vi "简易流程调试界面.vi"() -> ()   [LabVIEW 2016, in "斯坦道氟化物.lvlib"]
uses:
  <vilib>/Utility/miscctls.llb/LVPointTypeDef.ctl
  <userlib>/_OpenG.lib/array/array.llb/Sort 1D Array (I32)__ogtk.vi
  <vilib>/Plasmionique/MB Master/MB_Master/MB_Master.lvclass
panel:
  in  "调试控件":enum32{"填充流程", "清洗流程", "测试流程", "排空流程", "其他流程"}(tab)
  in  "填充简易流程":i32(listbox)
  in  "清洗简易流程":i32(listbox)
  in  "测试简易流程":i32(listbox)
  in  "排空简易流程":i32(listbox)
  in  "其他简易流程":i32(listbox)
  in  "停止":bool
  in  "单步测试":bool
  out "注射器温度":sgl
  out "消解温度":sgl
  out "ADC":sgl
  out "F3":sgl format="%#.6f"
  out "F2":sgl format="%#.6f"
  out "F1":sgl format="%#.6f"
  out "F0":sgl format="%#.6f"
  in  "启动":bool
  in  "参数下拉列表":u16(ring) items=["总氮"=2]
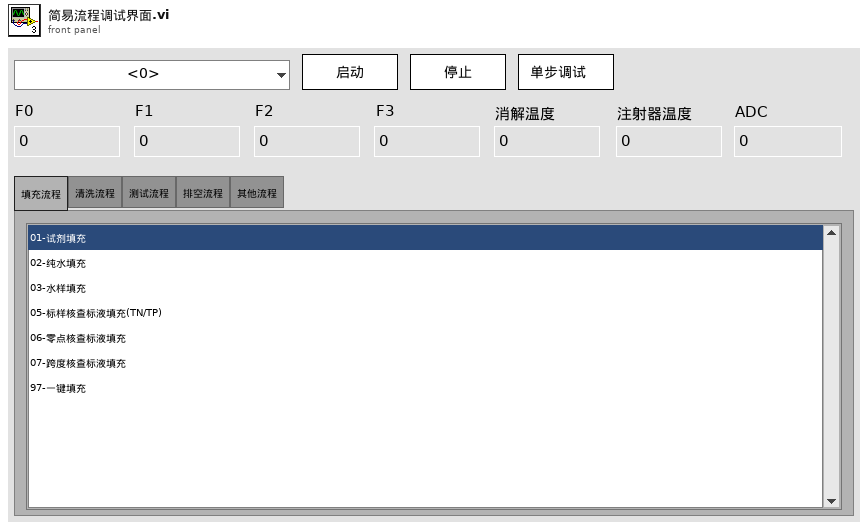
[diagram p1: front panel]
types:
  T1 = typedef "LVPointTypeDef.ctl" = cluster{"Horizontal":i16, "Vertical":i16}
  T2 = typedef "LVRectTypeDef.ctl" = cluster{"Left":i16, "Top":i16, "Right":i16, "Bottom":i16}
  T3 = typedef "LVStringsAndValuesArrayTypeDef_U16.ctl" = cluster{"String":string, "Value":u16}[]
  T4 = typedef "操作日志字段定义.ctl" = cluster{"时间":timestamp, "参数":string, "日志信息":string, "流程参数":string}
  T5 = enum16{"跨度核查", "水样测量", "零点核查", "标样核查", "加标回收", "快捷测试", "空白校准", "标样校准"}
  T6 = cluster{"系统时间":timestamp, "工作状态":u16, "测量模式":enum16{"待机", "连续模式", "周期模式", "定点模式", "受控模式", "手动模式"}, "告警代码":u16, "故障代码":u16, "日志代码":u16, "软件版本":u16, "F0":sgl, "F1":sgl, "F2":sgl, "F3":sgl, "T":sgl, "H":sgl, "id":u16, "flowid":u16, "量程":u16, "总磷控温温度1":sgl, "营养盐控温温度2":sgl, "ADC":sgl}
  T7 = enum32{"Bad", "Idle", "Run top level", "Running"}
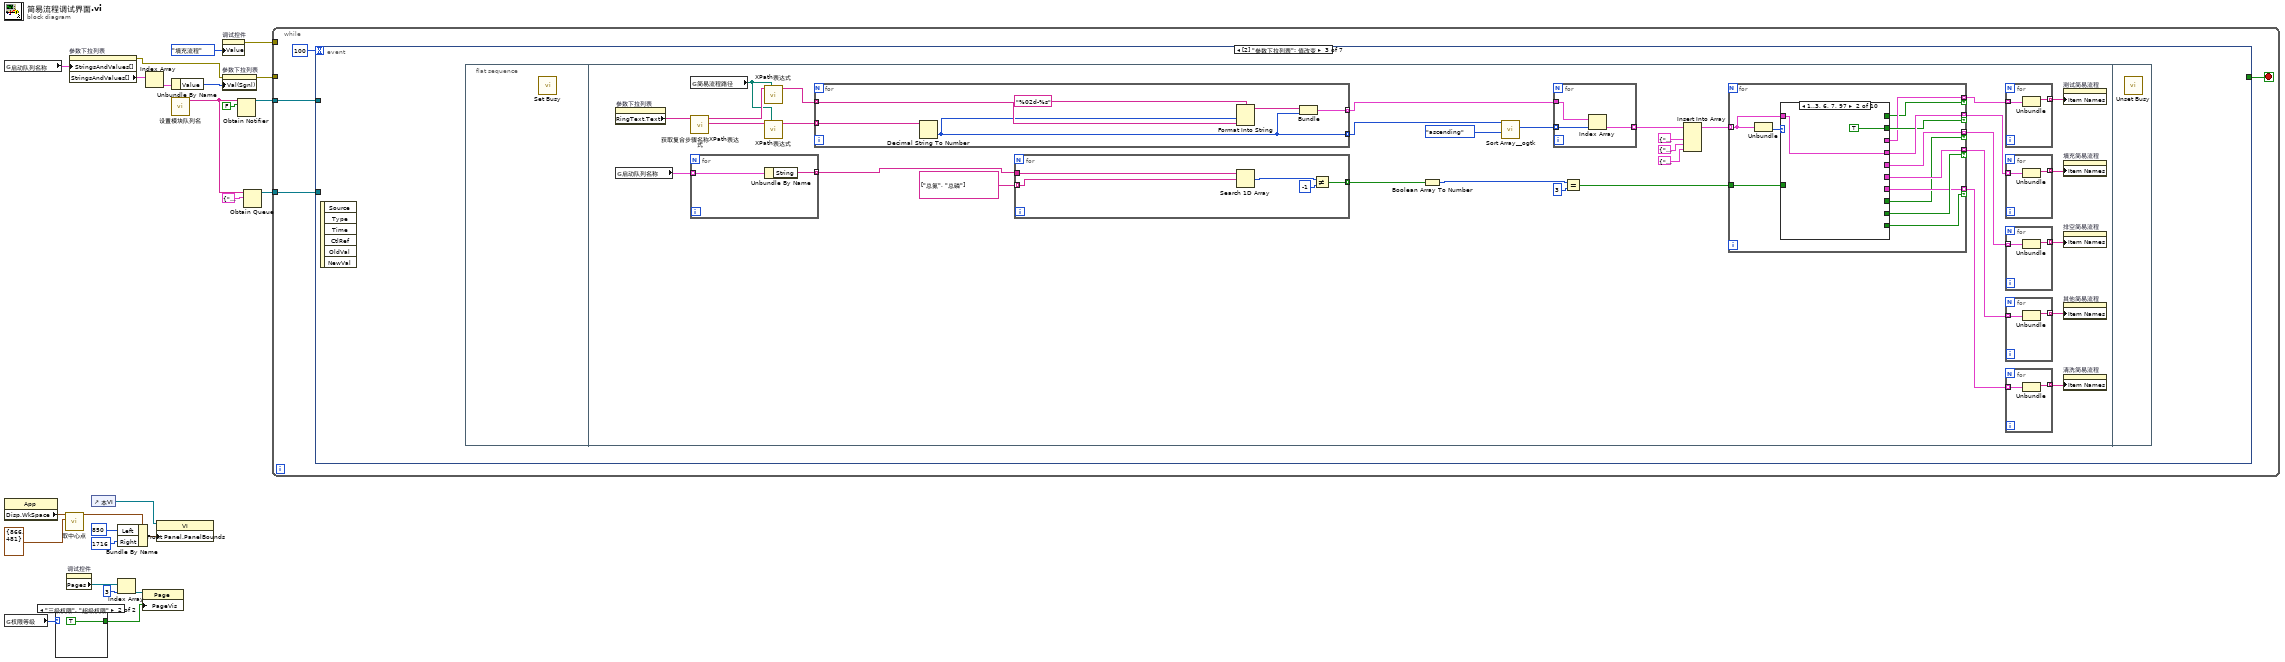
[diagram p0: block diagram]
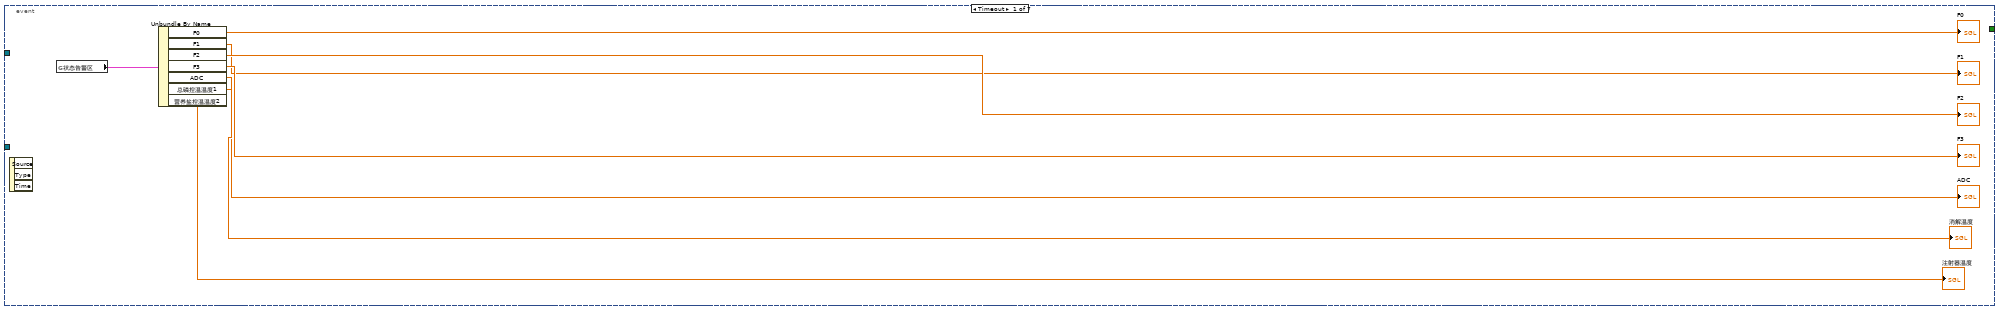
[diagram p3: hidden frame]
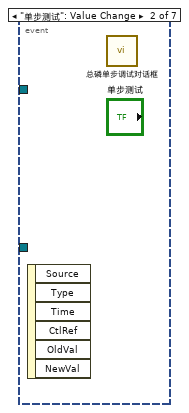
[diagram p4: hidden frame]
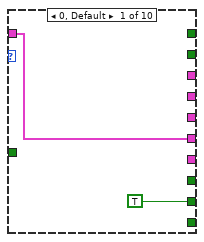
[diagram p5: hidden frame]
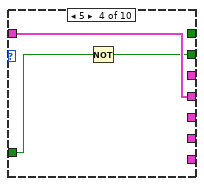
[diagram p7: hidden frame]
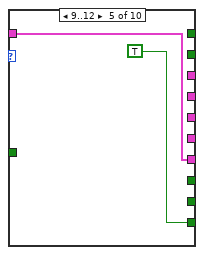
[diagram p8: hidden frame]
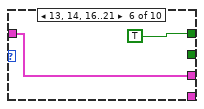
[diagram p9: hidden frame]
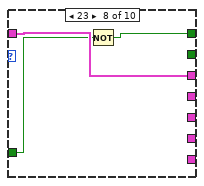
[diagram p11: hidden frame]
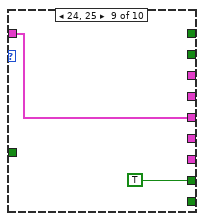
[diagram p12: hidden frame]
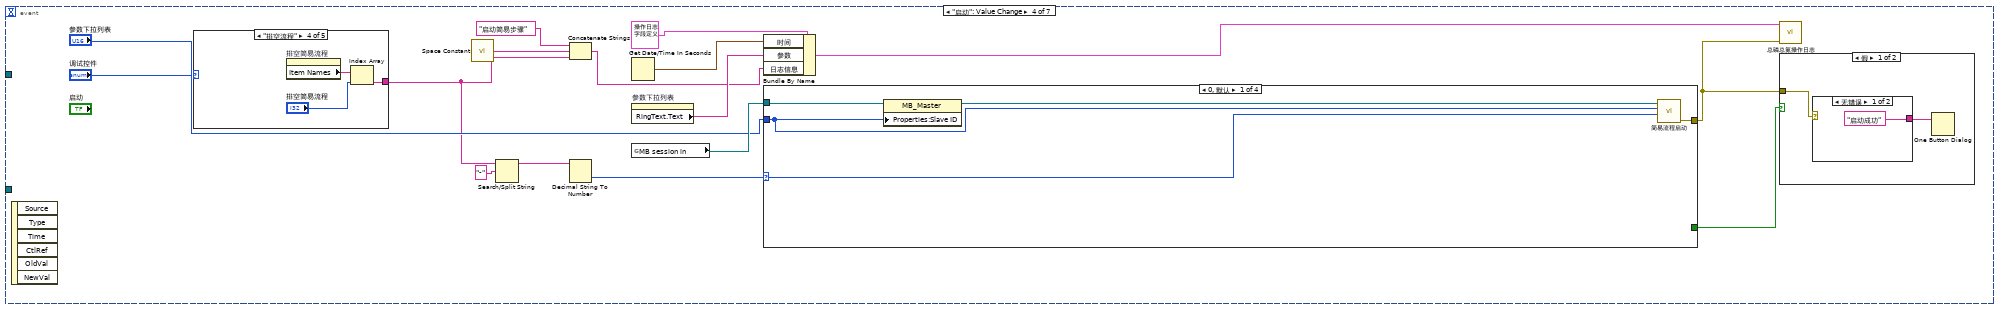
[diagram p14: hidden frame]
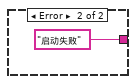
[diagram p15: hidden frame]
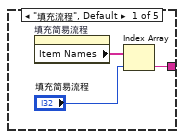
[diagram p17: hidden frame]
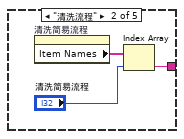
[diagram p18: hidden frame]
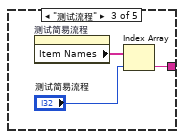
[diagram p19: hidden frame]
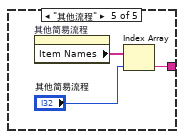
[diagram p20: hidden frame]
diagram:
  n1 = global read "model config var.vi" "启动队列名称"() -> (w20:cluster{"String":string, "Value":u16}[])
  n2 = property class="App"() -> ("Disp.WkSpace"=w6:T2)  [unwired: 2 in, 2 out]
  n3 = global read "VAR总磷总氮全局变量.vi" "权限等级"() -> (w12:enum16{"一级权限", "二级权限", "三级权限", "超级权限"})
  n4 = case shown="\"三级权限\", \"超级权限\"" w12 {
    tunnel: [_ TRUE ("选项卡可见")] -> w8
    frame "一级权限", Default {
    }
    frame "三级权限", "超级权限" {
    }
  }
  n5 = call "取中心点.vi"("前面板窗口:最小尺寸"=T1 {"Horizontal"=866, "Vertical"=481}, "显示:主工作区"=w6) -> ("前面板窗口:窗口边界"=w4:T2)  [unwired: 9 in]
  n6 = property on="调试控件" class="TabCtl (严格)"() -> ("Pages"=w11:refnum<vi>[])  [unwired: 2 in, 2 out]
  n7 = property on="参数下拉列表" class="Ring (严格)"("StringsAndValues[]"=w20) -> (error out=w21:errorcluster, "StringsAndValues[]"=w24:T3)  [unwired: 2 in, 1 out]
  n8 = control-ref of="本VI"() -> (w7:refnum<vi>)
  n9 = Bundle By Name(cluster=w4, "Left"=i16 850, "Right"=i16 1716) -> (w3:T2)
  n10 = Index Array(array=w11, index=3 ("索引")) -> (element=w9:refnum<vi>)
  n11 = property class="Page"(reference=w9, "PageVis"=w8) -> ()  [unwired: 1 in, 2 out]
  n12 = Index Array(array=w24) -> (element=w23:cluster{"String":string, "Value":u16})  [unwired: 1 in]
  n13 = property class="VI"(reference=w7, "Front Panel.PanelBounds"=w3) -> ()  [unwired: 1 in, 2 out]
  n14 = Unbundle By Name(w23) -> ("Value"=w22:u16)
  n15 = call "设置模块队列名.vi"() -> ("Msg"=w17:string)  [unwired: 5 in]
  n16 = property on="调试控件" class="TabCtl (严格)"("Value"=enum32{"填充流程", "清洗流程", "测试流程", "排空流程", "其他流程"}."填充流程" ("调试控件")) -> (error out=w13:errorcluster)  [unwired: 2 in, 1 out]
  n17 = property on="参数下拉列表" class="Ring (严格)"(error in=w21, "Val(Sgnl)"=w22) -> (error out=w25:errorcluster)  [unwired: 1 in, 1 out]
  n18 = Obtain Notifier(name (unnamed)=w17, notification data type=FALSE) -> (notifier out=w16:refnum<notifier>)  [unwired: 2 in, 2 out]
  n19 = Obtain Queue(name (unnamed)=w17, element data type=cluster{"命令":string, "data":variant} {"命令"="", "data"=variant}) -> (queue out=w15:refnum<queue>)  [unwired: 3 in, 2 out]
  n20 = while {
    tunnel: w25 -> [_]
    tunnel: w16 -> [w28]
    tunnel: w15 -> [w27]
    tunnel: w13 -> [_]
    stop <- w30 stop-if-true
    n21 = event shown="[2] \"参数下拉列表\": 值改变" {
      selector: _ -> [_ _ _ _ _ _ _]
      dyn-events: _ -> [_ _ _ _ _ _ _]
      timeout: 100 -> [_ _ _ _ _ _ _]
      tunnel: [_ _ _ _ _ _ TRUE] -> w30
      tunnel: w28 -> [_ _ _ _ _ w214 _]
      tunnel: w27 -> [_ _ _ _ _ w213 _]
      event Timeout {
        n22 = event-data() -> ()  [unwired: 1 in, 3 out]
        n23 = global read "VAR总磷总氮全局变量.vi" "状态告警区"() -> (w38:T6)
        n24 = Unbundle By Name(w38) -> ("F0"=→"F0":sgl, "F1"=→"F1":sgl, "F2"=→"F2":sgl, "F3"=→"F3":sgl, "ADC"=→"ADC":sgl, "总磷控温温度1"=→"消解温度":sgl, "营养盐控温温度2"=→"注射器温度":sgl)
      }
      event "单步测试": Value Change {
        n25 = event-data() -> ()  [unwired: 1 in, 6 out]
        n26 = call "总磷单步调试对话框.vi"() -> ()  [unwired: 12 in]
      }
      event "参数下拉列表": Value Change {
        n27 = event-data() -> ()  [unwired: 1 in, 6 out]
        n28 = flat-sequence {
          frame #0 {
            n29 = call <vilib>:"Set Busy.vi"() -> ()  [unwired: 10 in, 2 out]
          }
          frame #1 {
            n30 = property on="参数下拉列表" class="Ring (严格)"() -> ("RingText.Text"=w70:string)  [unwired: 2 in, 2 out]
            n31 = global read "model config var.vi" "启动队列名称"() -> (w45:cluster{"String":string, "Value":u16}[])
            n32 = global read "总磷总氮断电保存全局变量.vi" "简易流程路径"() -> (w65:path)
            n33 = call "获取复合步骤名称XPath表达式.vi"("查询参数"=w70) -> ("FlowId"=w68:string, "name"=w69:string)  [unwired: 9 in]
            n34 = for {
              tunnel: w45 -> [w72] mode=indexing
              tunnel: [w71] -> w44 mode=indexing
              n35 = Unbundle By Name(w72) -> ("String"=w71:string)
            }
            n36 = call "XPath表达式.vi"("添加的路径"=w65, "XPath expression"=w69) -> ("数组"=w67:string[])  [unwired: 9 in]
            n37 = call "XPath表达式.vi"("添加的路径"=w65, "XPath expression"=w68) -> ("数组"=w66:string[])  [unwired: 9 in]
            n38 = for {
              tunnel: w67 -> [w127] mode=indexing
              tunnel: w66 -> [w130] mode=indexing
              tunnel: [w129] -> w62 mode=indexing
              tunnel: [w125] -> w64 mode=indexing
              n39 = Decimal String To Number(string=w130) -> (number=w125:i32)  [unwired: 2 in, 1 out]
              n40 = Format Into String(format string="%02d-%s" ("格式字符串"), w125, w127) -> (resulting string=w126:string)  [unwired: 2 in, 1 out]
              n41 = Bundle(w126, w125) -> (w129:cluster{string, i32})  [unwired: 1 in]
            }
            n42 = for {
              tunnel: string[] ["总氮", "总磷"] -> [w76] mode=indexing
              tunnel: w44 -> [w77]
              tunnel: [w73] -> w43 mode=indexing
              n43 = Search 1D Array(1D array=w77, element=w76) -> (index of element=w75:i32)  [unwired: 1 in]
              n44 = Not Equal?(x=w75, y=-1) -> (x != y?=w73:bool)
            }
            n45 = Boolean Array To Number(Boolean array=w43) -> (number=w42:u32)
            n46 = call-poly <userlib>:"Sort Array__ogtk.vi"("Order"=enum16{"ascending", "descending"}."ascending", "Array in"=w64) -> ("Sorted Pointers"=w61:i32[])  [unwired: 8 in, 1 out]
            n47 = for {
              tunnel: w62 -> [w124]
              tunnel: w61 -> [w123] mode=indexing
              tunnel: [w122] -> w56 mode=indexing
              n48 = Index Array(array=w124, index=w123) -> (element=w122:cluster{string, i32})
            }
            n49 = Equal?(x=w42, y=u32 3) -> (x = y?=w40:bool)
            n50 = Insert Into Array(array=w56, new element #1=cluster{string, i32} {"97-一键填充", 97} ("新元素/子数组"), new element #2=cluster{string, i32} {"98-快捷测试（低量程）", 98} ("新元素/子数组"), new element #3=cluster{string, i32} {"99-快捷测试（高量程）", 99} ("新元素/子数组")) -> (w55:cluster{string, i32}[])  [unwired: 1 in]
            n51 = for {
              tunnel: w55 -> [w99] mode=indexing
              tunnel: [w98] -> w48 mode=indexing if=w97
              tunnel: [w96] -> w58 mode=indexing if=w95
              tunnel: [w94] -> w54 mode=indexing if=w93
              tunnel: [w92] -> w52 mode=indexing if=w91
              tunnel: [w90] -> w50 mode=indexing if=w89
              tunnel: w40 -> [w88]
              n52 = Unbundle(w99) -> (w100:i32)  [unwired: 1 out]
              n53 = case shown="1..3, 6, 7, 97" w100 {
                tunnel: [w102 _ _ _ _ _ _ _ _ _] -> w98
                tunnel: w99 -> [w102 w104 w106 w109 w111 w113 w115 w118 w120 w121]
                tunnel: [TRUE _ _ _ _ _ _ _ _ _] -> w97
                tunnel: [_ w104 w106 w109 _ _ _ _ _ _] -> w96
                tunnel: [_ TRUE w105 w107 _ _ _ _ _ _] -> w95
                tunnel: [_ _ _ _ w111 _ _ _ _ _] -> w94
                tunnel: [_ _ _ _ TRUE _ _ _ _ _] -> w93
                tunnel: [_ _ _ _ _ w113 w115 w118 _ _] -> w92
                tunnel: [_ _ _ _ _ TRUE w114 w116 _ _] -> w91
                tunnel: [_ _ _ _ _ _ _ _ w120 w121] -> w90
                tunnel: [_ _ _ _ _ _ _ _ TRUE _] -> w89
                tunnel: w88 -> [_ _ w105 w108 _ _ w114 w117 _ _]
                frame 0, Default {
                }
                frame 1..3, 6, 7, 97 {
                }
                frame 4 {
                }
                frame 5 {
                  n54 = Not(x=w108) -> (.not. x?=w107:bool)
                }
                frame 9..12 {
                }
                frame 13, 14, 16..21 {
                }
                frame 22 {
                }
                frame 23 {
                  n55 = Not(x=w117) -> (.not. x?=w116:bool)
                }
                frame 24, 25 {
                }
                frame 8, 15 {
                }
              }
            }
            n56 = for {
              tunnel: w52 -> [w83] mode=indexing
              tunnel: [w82] -> w51 mode=indexing
              n57 = Unbundle(w83) -> (w82:string)  [unwired: 1 out]
            }
            n58 = for {
              tunnel: w58 -> [w87] mode=indexing
              tunnel: [w86] -> w57 mode=indexing
              n59 = Unbundle(w87) -> (w86:string)  [unwired: 1 out]
            }
            n60 = for {
              tunnel: w50 -> [w81] mode=indexing
              tunnel: [w80] -> w49 mode=indexing
              n61 = Unbundle(w81) -> (w80:string)  [unwired: 1 out]
            }
            n62 = for {
              tunnel: w48 -> [w79] mode=indexing
              tunnel: [w78] -> w47 mode=indexing
              n63 = Unbundle(w79) -> (w78:string)  [unwired: 1 out]
            }
            n64 = for {
              tunnel: w54 -> [w85] mode=indexing
              tunnel: [w84] -> w53 mode=indexing
              n65 = Unbundle(w85) -> (w84:string)  [unwired: 1 out]
            }
            n66 = property on="测试简易流程" class="LstBox (严格)"("Item Names"=w51) -> ()  [unwired: 2 in, 2 out]
            n67 = property on="填充简易流程" class="LstBox (严格)"("Item Names"=w57) -> ()  [unwired: 2 in, 2 out]
            n68 = property on="排空简易流程" class="LstBox (严格)"("Item Names"=w49) -> ()  [unwired: 2 in, 2 out]
            n69 = property on="其他简易流程" class="LstBox (严格)"("Item Names"=w47) -> ()  [unwired: 2 in, 2 out]
            n70 = property on="清洗简易流程" class="LstBox (严格)"("Item Names"=w53) -> ()  [unwired: 2 in, 2 out]
          }
          frame #2 {
            n71 = call <vilib>:"Unset Busy.vi"() -> ()  [unwired: 11 in, 1 out]
          }
        }
      }
      event "启动": Value Change {
        n72 = event-data() -> ()  [unwired: 1 in, 6 out]
        n73 = case shown="\"排空流程\"" "调试控件" {
          tunnel: [w151 w154 w157 w160 w163] -> w132
          frame "填充流程", Default {
            n74 = property on="填充简易流程" class="LstBox (严格)"() -> ("Item Names"=w153:string[])  [unwired: 2 in, 2 out]
            n75 = Index Array(array=w153, index="填充简易流程") -> (element=w151:string)
          }
          frame "清洗流程" {
            n76 = property on="清洗简易流程" class="LstBox (严格)"() -> ("Item Names"=w156:string[])  [unwired: 2 in, 2 out]
            n77 = Index Array(array=w156, index="清洗简易流程") -> (element=w154:string)
          }
          frame "测试流程" {
            n78 = property on="测试简易流程" class="LstBox (严格)"() -> ("Item Names"=w159:string[])  [unwired: 2 in, 2 out]
            n79 = Index Array(array=w159, index="测试简易流程") -> (element=w157:string)
          }
          frame "排空流程" {
            n80 = property on="排空简易流程" class="LstBox (严格)"() -> ("Item Names"=w162:string[])  [unwired: 2 in, 2 out]
            n81 = Index Array(array=w162, index="排空简易流程") -> (element=w160:string)
          }
          frame "其他流程" {
            n82 = property on="其他简易流程" class="LstBox (严格)"() -> ("Item Names"=w165:string[])  [unwired: 2 in, 2 out]
            n83 = Index Array(array=w165, index="其他简易流程") -> (element=w163:string)
          }
        }
        n84 = call <vilib>:"Space Constant.vi"() -> ("String"=w131:string)
        n85 = Search/Split String(string=w132, search string/char (-)="-" ("搜索字符串/字符(-)")) -> (substring before match=w142:string)  [unwired: 1 in, 2 out]
        n86 = Concatenate Strings("启动简易步骤" ("日志信息"), w131, w132) -> (w133:string)
        n87 = Decimal String To Number(string=w142) -> (number=w141:i32)  [unwired: 2 in, 1 out]
        n88 = Get Date/Time In Seconds() -> (seconds since 1Jan1904=w137:timestamp)
        n89 = property on="参数下拉列表" class="Ring (严格)"() -> ("RingText.Text"=w136:string)  [unwired: 2 in, 2 out]
        n90 = global read "VAR总磷总氮全局变量.vi" "MB session in"() -> (w146:refnum<class "MB_Master.lvclass">)
        n91 = Bundle By Name(cluster=T4 {"时间"=timestamp(0 s since 1904-01-01), "参数"="", "日志信息"="", "流程参数"=""} ("data in"), "时间"=w137, "参数"=w136, "日志信息"=w133) -> (w138:T4)
        n92 = case shown="0, 默认" w141 {
          selector: w141 -> [w168 w179 _ w200]
          tunnel: [w170 w180 _ w204] -> w134
          tunnel: w146 -> [w167 w178 _ w203]
          tunnel: "参数下拉列表" -> [w166 w177 w186 w202]
          tunnel: [_ w176 _ _] -> w140
          frame 0, Default {
            n93 = property class="MB_Master"(reference=w167, "Properties:Slave ID"=w166) -> (reference out=w169:refnum<class "MB_Master.lvclass">)  [unwired: 1 in, 1 out]
            n94 = call "简易流程启动.vi"("简易流程"=w168, "参数Id"=w166, "MB session in"=w169) -> ("error out"=w170:errorcluster)  [unwired: 7 in, 1 out]
          }
          frame 24 {
            n95 = call "警示对话框.vi"("副标题颜色"=u32 0, "主标题颜色"=u32 16711680, "副标题"="请确认所有试剂均已拆除，除纯水管外所有管路接入废液桶（瓶）！" ("消息"), "主标题"="警告！！！" ("消息")) -> ("check"=w171:bool)  [unwired: 7 in]
            n96 = Not(x=w171) -> (.not. x?=w176:bool)
            n97 = case shown="真" w171 {
              tunnel: [_ w185] -> w180
              tunnel: w179 -> [_ w183]
              tunnel: w178 -> [_ w182]
              tunnel: w177 -> [_ w181]
              frame False {
              }
              frame True {
                n98 = property class="MB_Master"(reference=w182, "Properties:Slave ID"=w181) -> (reference out=w184:refnum<class "MB_Master.lvclass">)  [unwired: 1 in, 1 out]
                n99 = call "简易流程启动.vi"("简易流程"=w183, "参数Id"=w181, "MB session in"=w184) -> ("error out"=w185:errorcluster)  [unwired: 7 in, 1 out]
              }
            }
          }
          frame 97 {
            n100 = vi-ref "一键清洗流程.vi"() -> (w187:refnum<vi>)
            n101 = property class="VI"(reference=w187) -> ("Name"=w188:string, "Exec.State"=w189:T7)  [unwired: 1 in, 2 out]
            n102 = case shown="\"Idle\"" w189 {
              tunnel: w188 -> [_ w198]
              tunnel: w186 -> [_ w191]
              frame "Bad", Default {
              }
              frame "Idle" {
                n103 = Open VI Reference(type specifier VI Refnum (for type only)=refnum<vi> refnum, vi path=w198, options=128 ("选项")) -> (vi reference=w195:refnum<vi>, error out=w193:errorcluster)  [unwired: 3 in]
                n104 = property on="填充简易流程" class="LstBox (严格)"() -> ("Item Names"=w190:string[])  [unwired: 2 in, 2 out]
                n105 = call-by-ref "开始异步调用"(reference=w195, error in=w193, "项名"=w190, "参数下拉列表"=w191) -> (reference out=w194:refnum<vi>, error out=w192:errorcluster)  [unwired: 10 in]
                n106 = Close Reference(reference=w194, error in (no error)=w192) -> ()  [unwired: 1 out]
              }
            }
          }
          frame 98, 99 {
            n107 = case shown="98, 默认" w200 {
              tunnel: [enum16{"低量程", "高量程"}."低量程" ("量程下拉列表") enum16{"低量程", "高量程"}."高量程" ("量程下拉列表")] -> w199
              frame 98, Default {
              }
              frame 99 {
              }
            }
            n108 = call "非国标启动命令.vi"("参数下拉列表"=w202, "量程下拉列表"=w199, "测量模式"=T5."快捷测试", "MB session in"=w203) -> ("error out"=w204:errorcluster)  [unwired: 6 in, 1 out]
          }
        }
        n109 = call "总磷总氮操作日志.vi"("错误输入（无错误）"=w134, "data in"=w138) -> ()  [unwired: 9 in, 1 out]
        n110 = case shown="假" w140 {
          tunnel: w134 -> [w148 _]
          frame False {
            n111 = case shown="无错误" w148 {
              tunnel: ["启动成功" "启动失败"] -> w147
              frame No Error {
              }
              frame Error {
              }
            }
            n112 = One Button Dialog(message=w147) -> ()  [unwired: 1 in, 1 out]
          }
          frame True {
          }
        }
      }
      event "排空简易流程": Mouse Down {
        n113 = event-data() -> ()  [unwired: 1 in, 6 out]
      }
      event "停止": Value Change {
        n114 = event-data() -> ()  [unwired: 1 in, 6 out]
        n115 = Get Date/Time In Seconds() -> (seconds since 1Jan1904=w210:timestamp)
        n116 = property on="参数下拉列表" class="Ring (严格)"() -> ("RingText.Text"=w207:string)  [unwired: 2 in, 2 out]
        n117 = Send Notification(notification=TRUE ("通知"), notifier=w214) -> ()  [unwired: 1 in, 2 out]
        n118 = Bundle By Name(cluster=T4 {"时间"=timestamp(0 s since 1904-01-01), "参数"="", "日志信息"="", "流程参数"=""} ("data in"), "时间"=w210, "参数"=w207, "日志信息"="手动停止") -> (w211:T4)
        n119 = Enqueue Element(queue=w213, element=cluster{"命令":string, "data":variant} {"命令"="启动", "data"=variant(cluster{"站号":u16, "控制命令输出":u16[]} {"站号"=1, "控制命令输出"=[2816]})} ("元素")) -> (queue out=w216:refnum<queue>)  [unwired: 2 in, 2 out]
        n120 = Enqueue Element(queue=w216, element=cluster{"命令":string, "data":variant} {"命令"="启动", "data"=variant(cluster{"站号":u16, "控制命令输出":u16[]} {"站号"=2, "控制命令输出"=[2816]})} ("元素")) -> (error out=w208:errorcluster)  [unwired: 2 in, 2 out]
        n121 = call "总磷总氮操作日志.vi"("错误输入（无错误）"=w208, "data in"=w211) -> ()  [unwired: 9 in, 1 out]
      }
      event Panel Close {
        n122 = event-data() -> ()  [unwired: 1 in, 3 out]
      }
    }
  }
